vi "Player Info.vi"(11 "Random in":refnum<class "Random.lvclass">) -> (0 "Defeat Speech":string, 1 "Victory Speech":string, 2 "Name":string, 3 "Random out":refnum<class "Random.lvclass">)   [LabVIEW 2015, in "Random.lvclass"]
uses:
  Random.lvclass
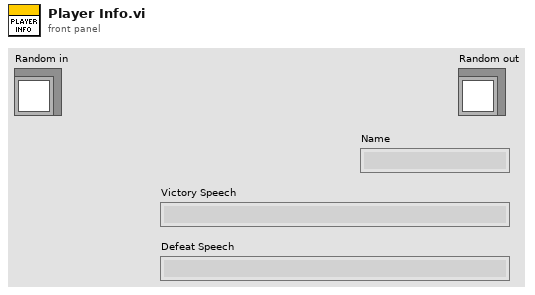
[diagram p1: front panel]
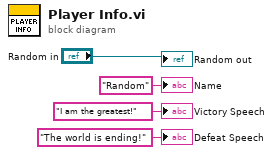
[diagram p0: block diagram]
diagram:
  "Random out" <- "Random in"
  "Name" <- "Random" ("Name")
  "Victory Speech" <- "I am the greatest!" ("Victory Speech")
  "Defeat Speech" <- "The world is ending!" ("Defeat Speech")
